vi "GEA2 Message Event Handler.vi"(4 "Data":refnum<user-event>, 5 "Event Data":T1, 6 "Control Ref":refnum<k24>, 7 "Event Common Data":T2) -> ()   [LabVIEW 2016, in "GEA2_Toolkit.lvlib"]
doc: "This subVI is executed upon receiving an event (GEA2 data). It parses the data and returns: source, destination, command, length, CRC, and data. The inputs CANNOT be modified."
uses:
  library/GEA2_Toolkit.lvlib
  type defs/Data Out.ctl
  C:/Technology Lab/NI-2010/Trunk/Utility/LabVIEW GEA2 Toolkit v1.0.0.0/Appliance.NET/GeaCommunication.dll
  Appliance.NET/GeaCommunication.dll
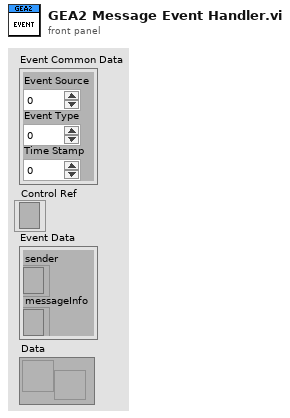
[diagram p1: front panel]
types:
  T1 = cluster{"sender":refnum<k24>, "messageInfo":refnum<k24>}
  T2 = cluster{"Event Source":i32, "Event Type":u32, "Time Stamp":u32}
  T3 = typedef "GEA2_Toolkit.lvlib/Data Out.ctl" = cluster{"Source":u8, "Destination":u8, "Command":u8, "Length":u8, "CRC":u16, "Message":string}
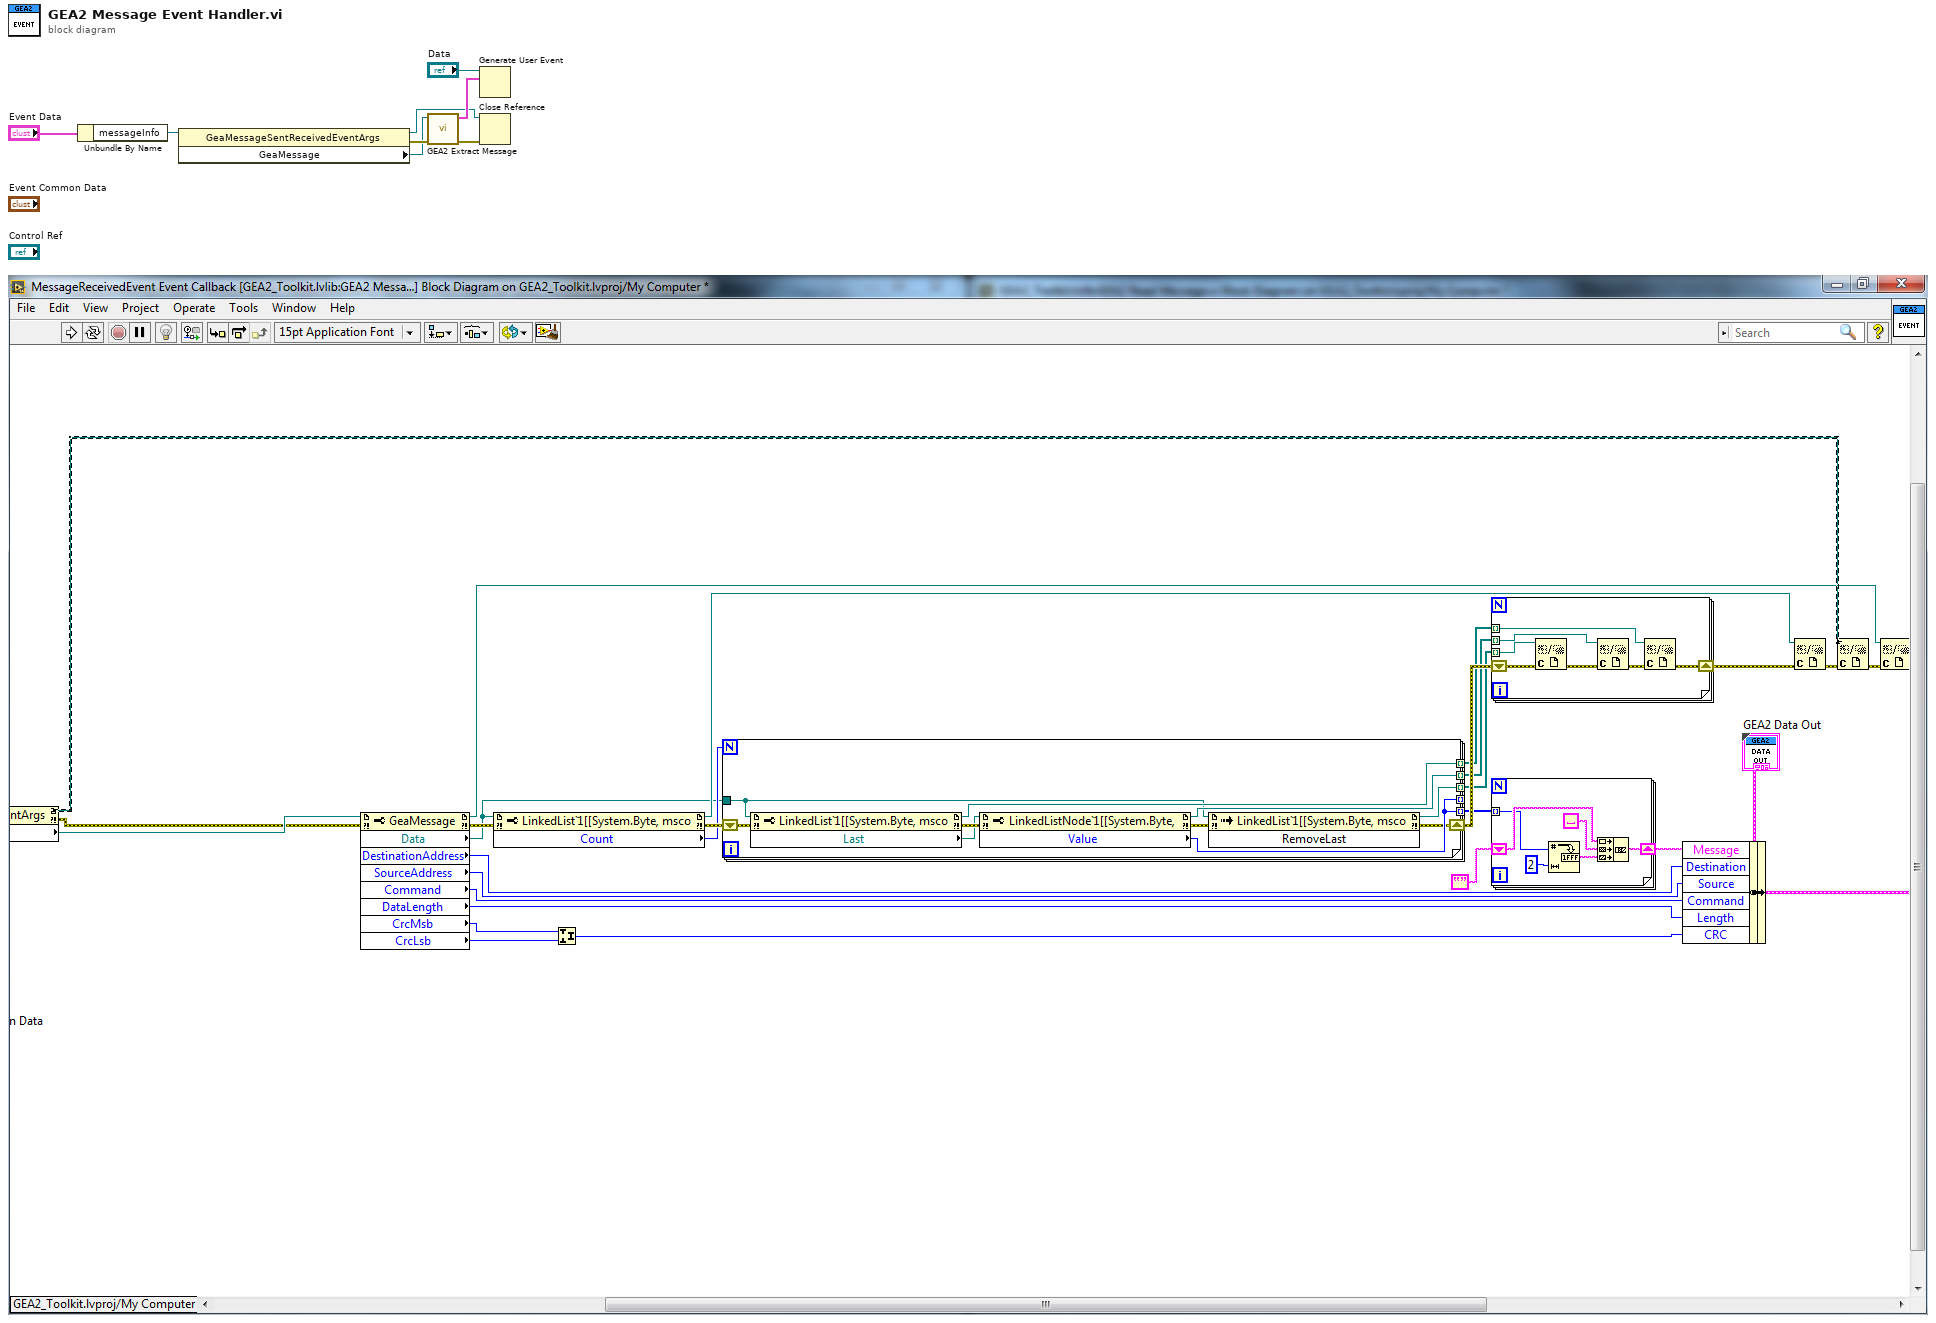
[diagram p0: block diagram]
diagram:
  n1 = Unbundle By Name("Event Data") -> ("messageInfo"=w3:refnum<k24>)
  n2 = property class="GeaMessageSentReceivedEventArgs"(reference=w3) -> (reference out=w4:refnum<k24>, error out=w7:errorcluster, "GeaMessage"=w6:refnum<k24>)  [unwired: 1 in]
  n3 = call "GEA2 Extract Message.vi"("error in (no error)"=w7, "GeaMessage"=w6) -> ("error out"=w1:errorcluster, "GEA2 Data Out"=w8:T3)  [unwired: 7 in, 1 out]
  n4 = Generate User Event(user event="Data", event data cluster=w8) -> ()  [unwired: 2 in, 2 out]
  n5 = Close Reference(reference=w4, error in (no error)=w1) -> ()  [unwired: 1 out]
